vi "PannelControl.vi"(7 "State":T1, 8 "에러 입력(에러 없음)":errorcluster) -> (0 "error out":errorcluster caption="에러 출력")   [LabVIEW 2019]
uses:
  03_Home/controller/pannelState.ctl
  globalValue.vi
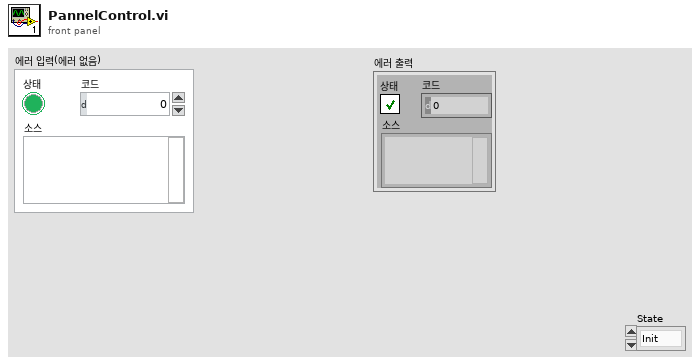
[diagram p1: front panel]
types:
  T1 = typedef "pannelState.ctl" = enum16{"Init", "LogIn", "SignUpView", "Home", "Management_patientList", "Management_patientTrashtList", "Management_patientCreate", "Management_patientUpdate", "Management_patientTraining", "Management_patientTrainingDetail", "H-MEDI PatientList", "H-MEDI HardwareCtl", "Adjust", "FineTuning", "UserList", "UserDetail", "Exit"}
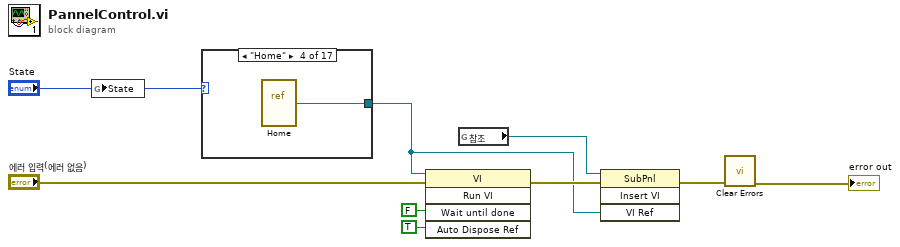
[diagram p0: block diagram]
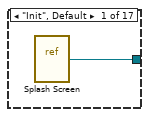
[diagram p2: hidden frame]
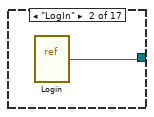
[diagram p3: hidden frame]
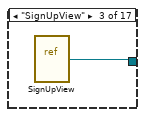
[diagram p4: hidden frame]
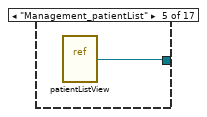
[diagram p5: hidden frame]
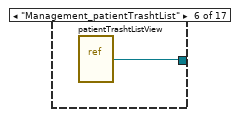
[diagram p6: hidden frame]
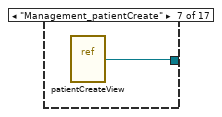
[diagram p7: hidden frame]
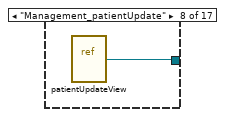
[diagram p8: hidden frame]
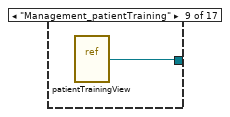
[diagram p9: hidden frame]
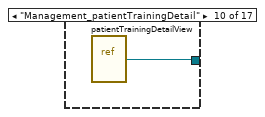
[diagram p10: hidden frame]
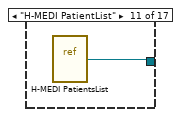
[diagram p11: hidden frame]
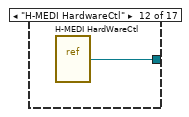
[diagram p12: hidden frame]
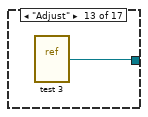
[diagram p13: hidden frame]
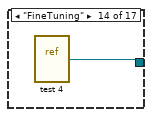
[diagram p14: hidden frame]
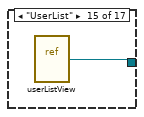
[diagram p15: hidden frame]
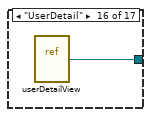
[diagram p16: hidden frame]
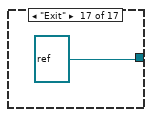
[diagram p17: hidden frame]
diagram:
  n1 = global write "globalValue.vi" "State"("State") -> ()
  n2 = case shown="\"Home\"" "State" {
    tunnel: [w10 w11 w12 w13 w14 w15 w16 w17 w18 w19 w20 w21 w22 w23 w24 w25 refnum<vi> refnum] -> w1
    frame "Init", Default {
      n3 = vi-ref "Splash Screen.vi"() -> (w10:refnum<vi>)
    }
    frame "LogIn" {
      n4 = vi-ref "Login.vi"() -> (w11:refnum<vi>)
    }
    frame "SignUpView" {
      n5 = vi-ref "SignUpView.vi"() -> (w12:refnum<vi>)
    }
    frame "Home" {
      n6 = vi-ref "Home.vi"() -> (w13:refnum<vi>)
    }
    frame "Management_patientList" {
      n7 = vi-ref "patientListView.vi"() -> (w14:refnum<vi>)
    }
    frame "Management_patientTrashtList" {
      n8 = vi-ref "patientTrashtListView.vi"() -> (w15:refnum<vi>)
    }
    frame "Management_patientCreate" {
      n9 = vi-ref "patientCreateView.vi"() -> (w16:refnum<vi>)
    }
    frame "Management_patientUpdate" {
      n10 = vi-ref "patientUpdateView.vi"() -> (w17:refnum<vi>)
    }
    frame "Management_patientTraining" {
      n11 = vi-ref "patientTrainingView.vi"() -> (w18:refnum<vi>)
    }
    frame "Management_patientTrainingDetail" {
      n12 = vi-ref "patientTrainingDetailView.vi"() -> (w19:refnum<vi>)
    }
    frame "H-MEDI PatientList" {
      n13 = vi-ref "H-MEDI PatientsList.vi"() -> (w20:refnum<vi>)
    }
    frame "H-MEDI HardwareCtl" {
      n14 = vi-ref "H-MEDI HardWareCtl.vi"() -> (w21:refnum<vi>)
    }
    frame "Adjust" {
      n15 = vi-ref "test 3.vi"() -> (w22:refnum<vi>)
    }
    frame "FineTuning" {
      n16 = vi-ref "test 4.vi"() -> (w23:refnum<vi>)
    }
    frame "UserList" {
      n17 = vi-ref "userListView.vi"() -> (w24:refnum<vi>)
    }
    frame "UserDetail" {
      n18 = vi-ref "userDetailView.vi"() -> (w25:refnum<vi>)
    }
    frame "Exit" {
    }
  }
  n19 = invoke class="VI" method="Run VI"(reference=w1, error in="에러 입력(에러 없음)", "Wait until done"=FALSE ("완료될 때까지 기다림"), "Auto Dispose Ref"=TRUE ("참조 자동 삭제")) -> (error out=w7:errorcluster)  [unwired: 1 in, 4 out]
  n20 = global read "globalValue.vi" "참조"() -> (w3:refnum<vi>)
  n21 = invoke class="SubPnl" method="Insert VI"(reference=w3, error in=w7, "VI Ref"=w1) -> (error out=w4:errorcluster)  [unwired: 1 in, 3 out]
  n22 = call <vilib>:"Clear Errors.vi"("error in (no error)"=w4) -> ("error out"=→"error out":errorcluster)  [unwired: 5 in, 1 out]
